vi "libssh2_channel_forward_listen.vi"(8 "error in (no error)":errorcluster, 10 "port in":i32, 11 "session":T2) -> (0 "error out":errorcluster, 2 "port out":i32, 3 "listener":T1)   [LabVIEW 2013, in "libssh2.lvlib"]
doc: "Create a listening channel for inbound TCP connections on a specific port on the SSH server. New connections are queued until accepted with <B>libssh2_channel_forward_accept</B>."
uses:
  libssh2.lvlib
  Session Refnum.ctl
  Listener Refnum.ctl
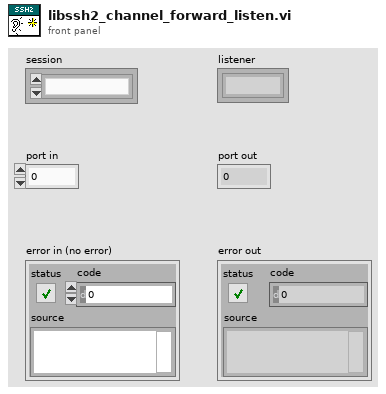
[diagram p1: front panel]
types:
  T1 = typedef "libssh2.lvlib/Listener Refnum.ctl" = refnum<k1>
  T2 = typedef "libssh2.lvlib/Session Refnum.ctl" = refnum<k1>
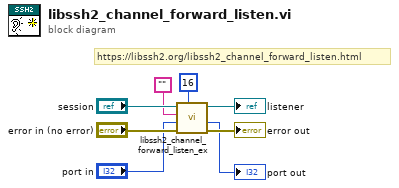
[diagram p0: block diagram]
diagram:
  # "https://libssh2.org/libssh2_channel_forward_listen.html"
  n1 = call "libssh2_channel_forward_listen_ex.vi"("queue_maxsize"=16, "error in (no error)"="error in (no error)", "port in"="port in", "host"="", "session"="session") -> ("error out"=→"error out":errorcluster, "port out"=→"port out":i32, "listener"=→"listener":T1)  [unwired: 4 in]
